vi "Fetch Multi Eval Meas IEM Margin Results.vi"(8 "error in (no error)":errorcluster, 9 "Result Type (Current)":i32(ring) items=["Current", "Average", "Extreme", "Standard Deviation"], 10 "Instance (1)":T2=1, 11 "VISA resource name":refnum<visa-resource-name>) -> (0 "error out":errorcluster, 1 "Margin Results":T1 {"Carrier Leakage" format="%^.3e"; "IQ Image" format="%^.3e"; "Margin" format="%^.3e"}, 2 "Reliability":i32, 3 "VISA resource name out":refnum<visa-resource-name>, 5 "Out Of Tolerance":i32)   [LabVIEW 2020, in "Rohde&Schwarz CMWXP NR FR1 Measurement.lvlib"]
doc: "Return the limit line margin results. The current margin indicates the minimum (vertical) distance between the inband emissions limit line and the current trace. A negative result indicates that the limit is exceeded. The average, extreme and standard deviation values are calculated from the current margins. The margin results cannot be displayed at the GUI.\n\nAttributes:\nRSCMWXPNRFR1M_ATTR_FETCH_MULTI_EVAL_MEAS_IEM_MARGIN_CURRENT_RESULTS\nRSCMWXPNRFR1M_ATTR_FETCH_MULTI_EVAL_MEAS_IEM_MARGIN_AVERAGE_RESULTS\nRSCMWXPNRFR1M_ATTR_FETCH_MULTI_EVAL_MEAS_IEM_MARGIN_EXTREME_RESULTS\nRSCMWXPNRFR1M_ATTR_FETCH_MULTI_EVAL_MEAS_IEM_MARGIN_STANDARD_DEVIATION_RESULTS\n\nRemote-control commands:\nFETCh:NRSub:MEAS<i>:MEValuation:IEMission:MARGin:CURRent?\nFETCh:NRSub:MEAS<i>:MEValuation:IEMission:MARGin:AVERage?\nFETCh:NRSub:MEAS<i>:MEValuation:IEMission:MARGin:EXTReme?\nFETCh:NRSub:MEAS<i>:MEValuation:IEMission:MARGin:SDEViation?"
uses:
  <instrlib>/Rohde&Schwarz CMWXP NR FR1 Measurement/Rohde&Schwarz CMWXP NR FR1 Measurement.lvlib
  <instrlib>/Rohde&Schwarz CMWXP NR FR1 Measurement/Private/_Instance.ctl
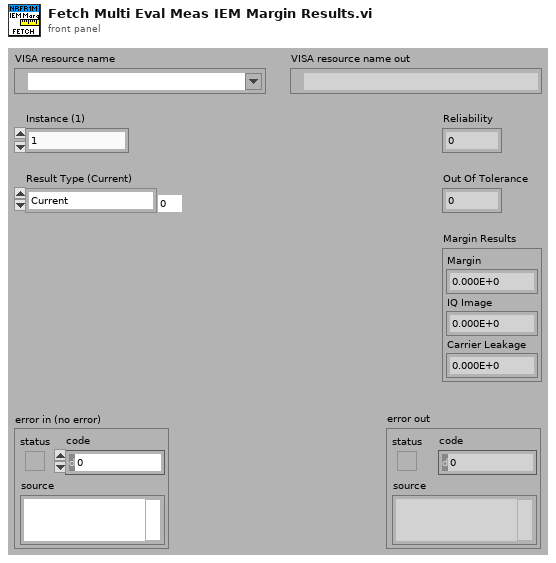
[diagram p1: front panel]
types:
  T1 = cluster{"Margin":dbl, "IQ Image":dbl, "Carrier Leakage":dbl}
  T2 = typedef "Rohde&Schwarz CMWXP NR FR1 Measurement.lvlib/_Instance.ctl" = i32
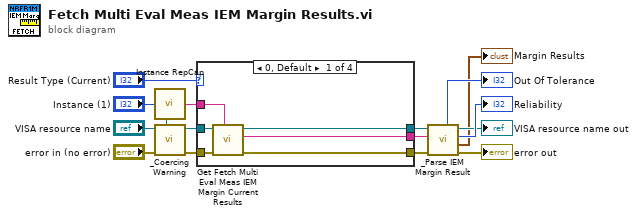
[diagram p0: block diagram]
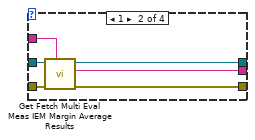
[diagram p2: hidden frame]
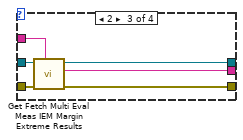
[diagram p3: hidden frame]
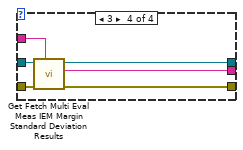
[diagram p4: hidden frame]
diagram:
  n1 = call <instrlib>:"Instance RepCap.vi"("Instance In"="Instance (1)") -> ("In Range?"=w13:bool, "RepCap Identifier Out"=w9:string)  [unwired: 1 in]
  n2 = call <instrlib>:"_Coercing Warning.vi"("In Range?"=w13, "error in (no error)"="error in (no error)", "VISA resource name"="VISA resource name") -> ("error out"=w11:errorcluster, "VISA resource name out"=w12:refnum<visa-resource-name>)  [unwired: 7 in]
  n3 = case shown="0, Default" "Result Type (Current)" {
    tunnel: w12 -> [w22 w28 w34 w40]
    tunnel: w11 -> [w21 w27 w33 w39]
    tunnel: [w20 w26 w32 w38] -> w6
    tunnel: w9 -> [w19 w25 w31 w37]
    tunnel: [w18 w24 w30 w36] -> w7
    tunnel: [w17 w23 w29 w35] -> w8
    frame 0, Default {
      n4 = call "Get Fetch Multi Eval Meas IEM Margin Current Results"("Repeated Capabilities"=w19, "error in (no error)"=w21, "instrument handle"=w22) -> ("error out"=w17:errorcluster, "Fetch Multi Eval Meas IEM Margin Current Results"=w18:string, "instrument handle out"=w20:refnum<visa-resource-name>)  [unwired: 6 in]
    }
    frame 1 {
      n5 = call "Get Fetch Multi Eval Meas IEM Margin Average Results"("Repeated Capabilities"=w25, "error in (no error)"=w27, "instrument handle"=w28) -> ("error out"=w23:errorcluster, "Fetch Multi Eval Meas IEM Margin Average Results"=w24:string, "instrument handle out"=w26:refnum<visa-resource-name>)  [unwired: 6 in]
    }
    frame 2 {
      n6 = call "Get Fetch Multi Eval Meas IEM Margin Extreme Results"("Repeated Capabilities"=w31, "error in (no error)"=w33, "instrument handle"=w34) -> ("error out"=w29:errorcluster, "Fetch Multi Eval Meas IEM Margin Extreme Results"=w30:string, "instrument handle out"=w32:refnum<visa-resource-name>)  [unwired: 6 in]
    }
    frame 3 {
      n7 = call "Get Fetch Multi Eval Meas IEM Margin Standard Deviation Results"("Repeated Capabilities"=w37, "error in (no error)"=w39, "instrument handle"=w40) -> ("error out"=w35:errorcluster, "Fetch Multi Eval Meas IEM Margin Standard Deviation Results"=w36:string, "instrument handle out"=w38:refnum<visa-resource-name>)  [unwired: 6 in]
    }
  }
  n8 = call <instrlib>:"_Parse IEM Margin Result.vi"("error in (no error)"=w8, "Input String"=w7, "VISA resource name"=w6) -> ("error out"=→"error out":errorcluster, "Margin Results"=→"Margin Results":T1, "Reliability"=→"Reliability":i32, "VISA resource name out"=→"VISA resource name out":refnum<visa-resource-name>, "Out Of Tolerance"=→"Out Of Tolerance":i32)  [unwired: 4 in]
